vi "Write Channel Map.vi"(8 "error in (no error)":errorcluster, 10 "Channel Map":map{string, T1}(c390), 11 "Zenoh in":refnum<class "Zenoh.lvclass">) -> (0 "error out":errorcluster, 3 "Zenoh out":refnum<class "Zenoh.lvclass">)   [LabVIEW 2021, in "Zenoh.lvclass"]
uses:
  Zenoh.lvclass
  Zenoh.lvclass/Zenoh.ctl
  typedef/Channel Info.ctl
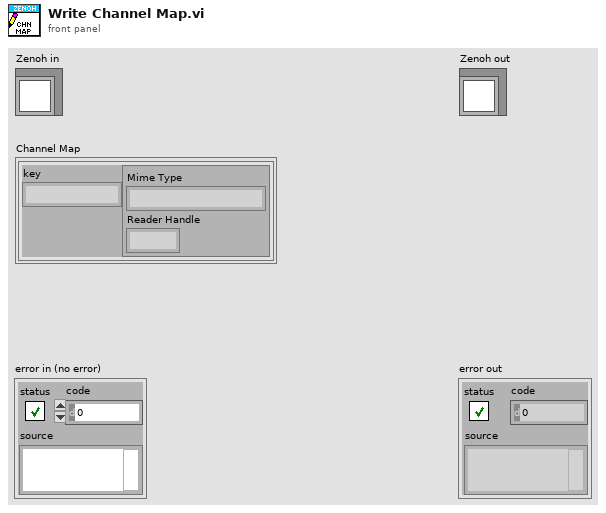
[diagram p1: front panel]
types:
  T1 = typedef "Zenoh.lvclass/Channel Info.ctl" = cluster{"Mime Type":string, "Reader Handle":u64}
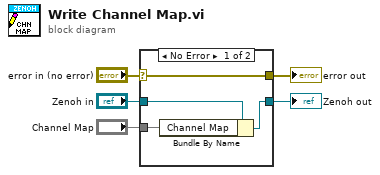
[diagram p0: block diagram]
diagram:
  n1 = case shown="No Error" "error in (no error)" {
    selector: "error in (no error)" -> [w9 w10]
    tunnel: [w9 w10] -> w4
    tunnel: [w7 w11] -> w2
    tunnel: "Zenoh in" -> [w8 w11]
    tunnel: "Channel Map" -> [w6 _]
    frame No Error {
      n2 = Bundle By Name(cluster=w8, "Channel Map"=w6) -> (w7:refnum<class "Zenoh.lvclass">)
    }
    frame Error {
    }
  }
  "error out" <- w4
  "Zenoh out" <- w2
